vi "Check For State.vi"(8 "error in (no error)":errorcluster, 10 "state":T1, 11 "Thread Manager in":refnum<class "Thread Manager.lvclass">) -> (0 "error out":errorcluster, 1 "private threads equal":bool[](array[boolean]), 2 "public threads equal":bool[](array[boolean]), 3 "Thread Manager out":refnum<class "Thread Manager.lvclass">)   [LabVIEW 2017, in "DSF Core.lvlib" / "Thread Manager.lvclass"]
uses:
  Thread Manager.lvclass
  Thread/Thread State.ctl
  Thread/Thread.lvclass
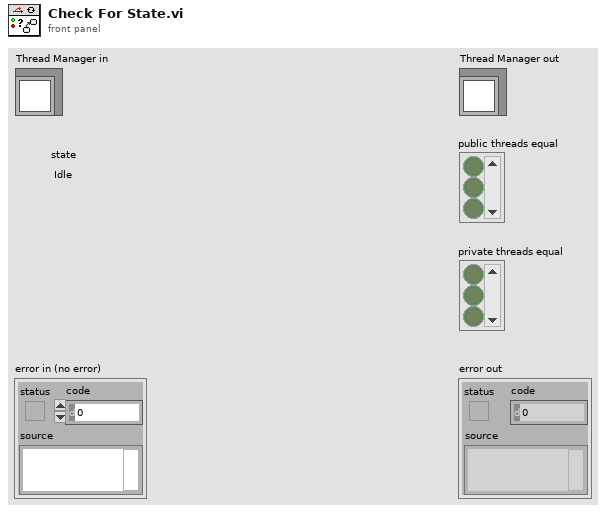
[diagram p1: front panel]
types:
  T1 = typedef "DSF Core.lvlib/Thread.lvclass/Thread State.ctl" = enum8{"Idle", "Running", "Error", "Shut Down"}
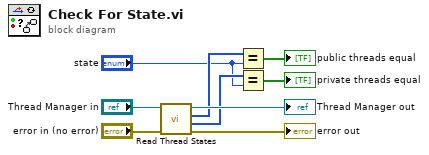
[diagram p0: block diagram]
diagram:
  n1 = call "Read Thread States.vi"("error in (no error)"="error in (no error)", "Thread Manager in"="Thread Manager in") -> ("error out"=→"error out":errorcluster, "private thread states"=w2:T1[], "public thread states"=w3:T1[], "Thread Manager out"=→"Thread Manager out":refnum<class "Thread Manager.lvclass">)  [unwired: 6 in]
  n2 = Equal?(x=w3, y="state") -> (x = y?=→"public threads equal":bool[])
  n3 = Equal?(x=w2, y="state") -> (x = y?=→"private threads equal":bool[])
